vi "Error Query.vi"(0 "VISA resource name":refnum<visa-resource-name>, 11 "error in (no error)":errorcluster) -> (4 "VISA resource name out":refnum<visa-resource-name>, 6 "Error Code":i32, 8 "Error Message":string, 15 "error out":errorcluster)   [LabVIEW 2020, in "eec 6700.lvlib"]
doc: "Queries the instrument for any errors in the instrument's error queue. It will continue to read errors until all errors have been read from the instrument. Any errors will be returned in the <B>error out</B> control.\n\n<B>Note:</B>\nThis VI is called automatically by most driver VIs so it is not usually necessary to call this in an application."
uses:
  <instrlib>/EEC6700LV-driver/eec 6700.lvlib
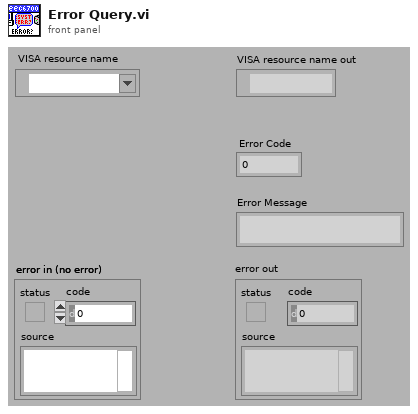
[diagram p1: front panel]
types:
  T1 = cluster{"Operation Complete":bool, "Not Used":bool, "Query Error":bool, "Device Error":bool, "Execution Error":bool, "Command Error":bool, "Not Used":bool, "Power On":bool}
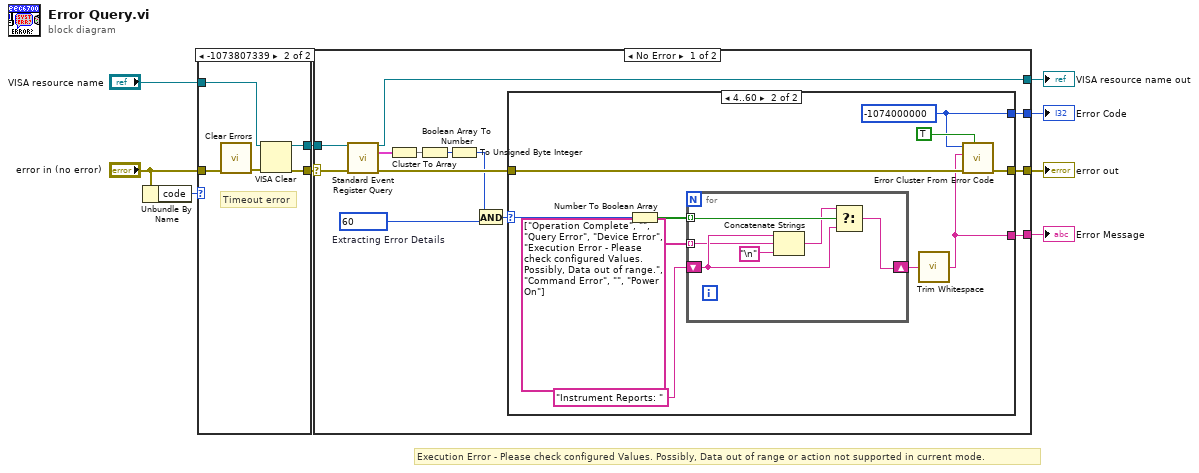
[diagram p0: block diagram]
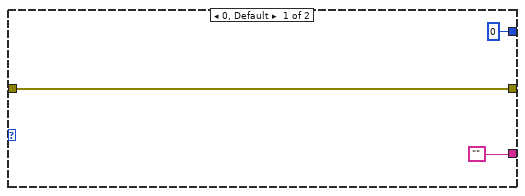
[diagram p2: hidden frame]
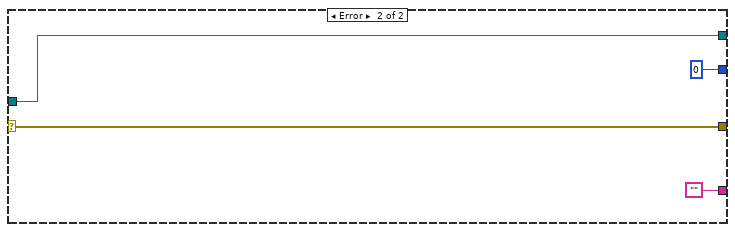
[diagram p3: hidden frame]
diagram:
  # "Execution Error - Please check configured Values. Possibly, Data out of range or action not supported in current mode."
  n1 = Unbundle By Name("error in (no error)") -> ("code"=w3:i32)
  n2 = case shown="-1073807339" w3 {
    tunnel: "error in (no error)" -> [w11 w16]
    tunnel: "VISA resource name" -> [w10 w14]
    tunnel: [w11 w12] -> w4
    tunnel: [w10 w15] -> w5
    frame Default {
    }
    frame -1073807339 {
      # "Timeout error"
      n3 = call <vilib>:"Clear Errors.vi"("error in (no error)"=w16) -> ("error out"=w13:errorcluster)  [unwired: 5 in, 1 out]
      n4 = VISA Clear(VISA resource name=w14, error in (no error)=w13) -> (VISA resource name out=w15:refnum<visa-resource-name>, error out=w12:errorcluster)
    }
  }
  n5 = case shown="No Error" w4 {
    selector: w4 -> [w22 w52]
    tunnel: [w29 w51] -> w9
    tunnel: [w28 w52] -> w8
    tunnel: w5 -> [w23 w51]
    tunnel: [w21 "" ("Empty String Constant")] -> w2
    tunnel: [w20 0 ("Code")] -> w1
    frame No Error {
      w26 = u8 60  # Extracting Error Details
      n6 = call <instrlib>:"Standard Event Register Query.vi"("VISA resource name"=w23, "error in (no error)"=w22) -> ("VISA resource name out"=w29:refnum<visa-resource-name>, "Standard Event Register"=w19:T1, "error out"=w27:errorcluster)  [unwired: 11 in]
      n7 = Cluster To Array(cluster=w19) -> (array=w17:bool[])
      n8 = Boolean Array To Number(Boolean array=w17) -> (number=w18:u32)
      n9 = To Unsigned Byte Integer(number=w18) -> (unsigned 8bit integer=w25:u8)
      n10 = And(x=w25, y=w26) -> (x .and. y?=w24:u8)
      n11 = case shown="4..60" w24 {
        selector: w24 -> [_ w36]
        tunnel: [w32 w35] -> w28
        tunnel: w27 -> [w32 w39]
        tunnel: ["" ("Empty String Constant") w34] -> w21
        tunnel: [0 ("Code") w33] -> w20
        frame 0, Default {
        }
        frame 4..60 {
          w33 = -1074000000 ("Code")
          n12 = Number To Boolean Array(number=w36) -> (Boolean array=w41:bool[])
          n13 = for {
            tunnel: w41 -> [w48] mode=indexing
            tunnel: string[] ["Operation Complete", "", "Query Error", "Device Error", "Execution Error - Please check configured Values. Possibly, Data out of range.", "Command Error", "", "Power On"] -> [w45] mode=indexing
            shift-right: [w47] -> w38
            shift-left: "Instrument Reports: " -> [w46]
            n14 = Concatenate Strings(w46, w45, "\n" ("Line Feed Constant")) -> (w44:string)
            n15 = Select(t=w44, s=w48, f=w46) -> (s? t:f=w47:string)
          }
          n16 = call <vilib>:"Trim Whitespace.vi"("string"=w38) -> ("trimmed string"=w34:string)  [unwired: 1 in]
          n17 = call <vilib>:"Error Cluster From Error Code.vi"("show call chain? (False)"=TRUE, "error in (no error)"=w39, "error message (\"\")"=w34, "error code (0)"=w33) -> ("error out"=w35:errorcluster)  [unwired: 5 in]
        }
      }
    }
    frame Error {
    }
  }
  "VISA resource name out" <- w9
  "error out" <- w8
  "Error Message" <- w2
  "Error Code" <- w1
